vi "PH_ImageCoG_Plotter.contents.vi"   [LabVIEW 2014, in "PH_ImageCoG_Plotter.lvlib"]
doc: "This class is forseen to operate on an image: it calculates the center of gravity. This class is connected to the class PH_ImageCalibrator which has to be used to produce a background image, and to the class PH_IEEE1394Camera to get an image from.\n\nThis class is part of the PHELIX user layer."
uses:
  PH_ImageCoG_Plotter.lvlib
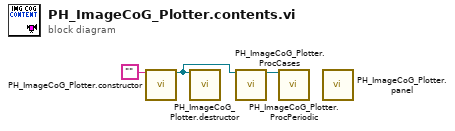
[diagram p0: block diagram]
diagram:
  n1 = call "PH_ImageCoG_Plotter.constructor.vi"("name"="") -> ("i ref out"=w1:refnum<vi>)  [unwired: 16 in, 2 out]
  n2 = call "PH_ImageCoG_Plotter.destructor.vi"("i ref in"=w1) -> ()  [unwired: 18 in, 1 out]
  n3 = call "PH_ImageCoG_Plotter.ProcCases.vi"("i ref in"=w1) -> ("i ref out"=w3:refnum<vi>)  [unwired: 16 in, 2 out]
  n4 = call "PH_ImageCoG_Plotter.ProcPeriodic.vi"("i ref in"=w3) -> ()  [unwired: 16 in, 3 out]
  n5 = call "PH_ImageCoG_Plotter.panel.vi"() -> ()  [unwired: 19 in, 1 out]
